vi "sort_points.vi"(8 "error in (no error)":errorcluster, 11 "TrajectoryDL120126ArbitraryLine2D in":refnum<class "TrajectoryDL120126ArbitraryLine2D.lvclass">=refnum) -> (0 "error out":errorcluster, 3 "TrajectoryDL120126ArbitraryLine2D out":refnum<class "TrajectoryDL120126ArbitraryLine2D.lvclass">)   [LabVIEW 2010, in "TrajectoryDL120126ArbitraryLine2D.lvclass"]
uses:
  TrajectoryDL120126ArbitraryLine2D.lvclass
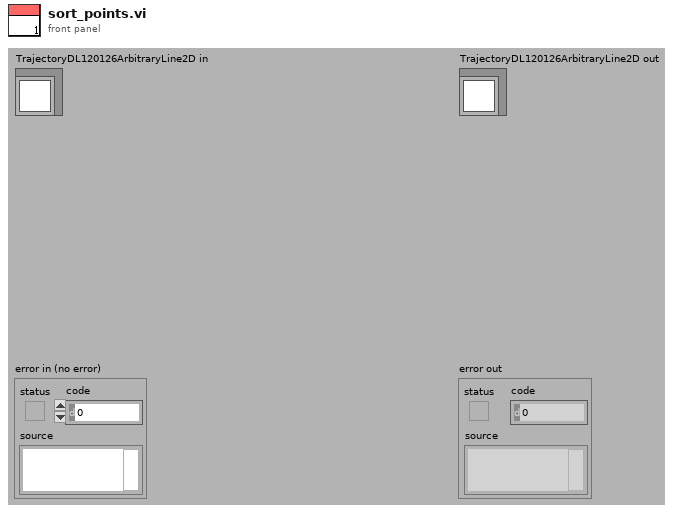
[diagram p1: front panel]
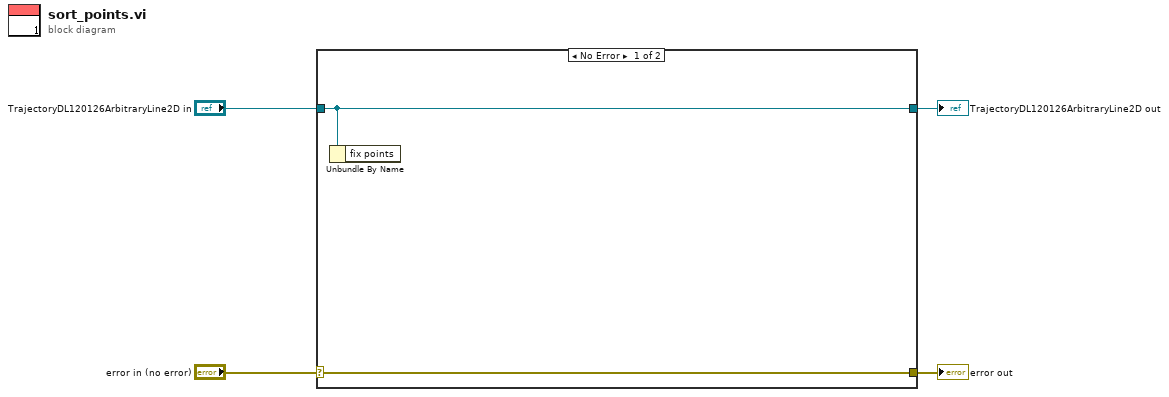
[diagram p0: block diagram]
diagram:
  n1 = case shown="No Error" "error in (no error)" {
    selector: "error in (no error)" -> [w6 w8]
    tunnel: [w6 w8] -> w3
    tunnel: [w5 w7] -> w1
    tunnel: "TrajectoryDL120126ArbitraryLine2D in" -> [w5 w7]
    frame No Error {
      n2 = Unbundle By Name(w5) -> ()  [unwired: 1 out]
    }
    frame Error {
    }
  }
  "error out" <- w3
  "TrajectoryDL120126ArbitraryLine2D out" <- w1
